vi "solar_app AppSetups (Dialog).vi"(11 "AppSetups":string[](array[string])) -> (3 "AppSetup":string)   [LabVIEW 2018]
doc: "This VI dialog selects the system setup to load for the application. Any setup other than \"Default\" adds a sub folder to the ..\\Configs folder. (i.e. \"Board\" Test Setup = ..\\Configs\\Board) All configuration files are kept in seperate folders for different system configurations."
panel:
  in  "Export":bool
  in  "OK":bool
  in  "Setup LB":i32(listbox)
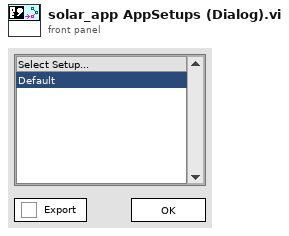
[diagram p1: front panel]
types:
  T1 = enum32{"invalid app kind", "Development System", "Run Time System", "Student Edition", "Embedded LabVIEW", "Evaluation", "Custom"}
  T2 = typedef "LVPoint32TypeDef.ctl" = cluster{"Horizontal":i32, "Vertical":i32}
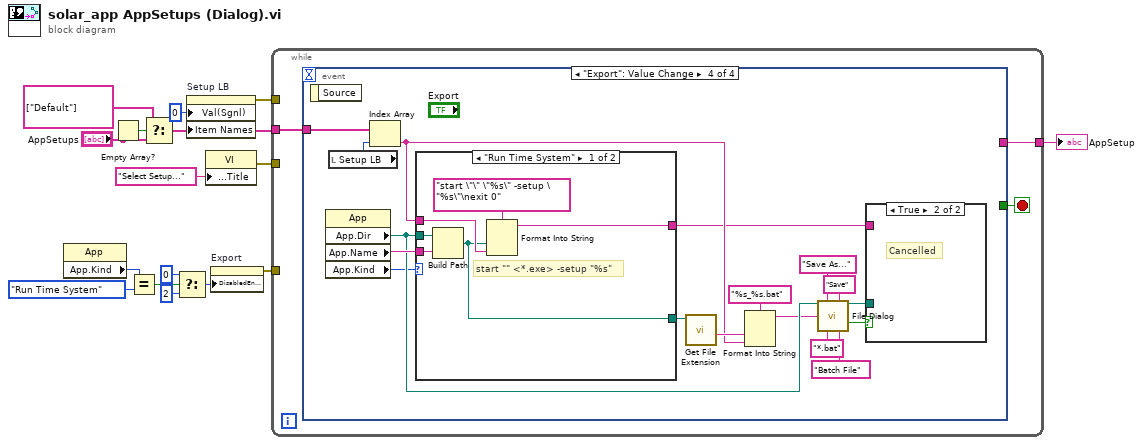
[diagram p0: block diagram]
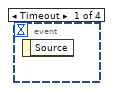
[diagram p2: hidden frame]
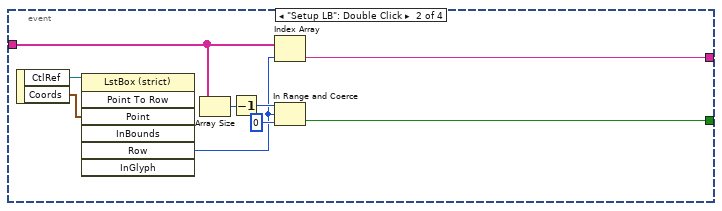
[diagram p3: hidden frame]
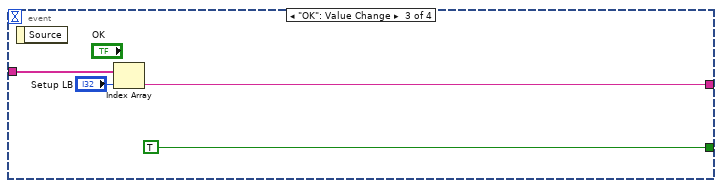
[diagram p4: hidden frame]
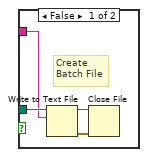
[diagram p5: hidden frame]
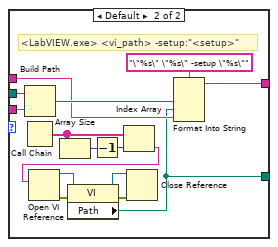
[diagram p6: hidden frame]
diagram:
  n1 = property class="App"() -> ("App.Kind"=w7:T1)  [unwired: 2 in, 2 out]
  n2 = Empty Array?(array="AppSetups") -> (empty?=w11:bool)
  n3 = Equal?(x=w7, y=T1."Run Time System") -> (x = y?=w5:bool)
  n4 = Select(t=string[] ["Default"], s=w11, f="AppSetups") -> (s? t:f=w8:string[])
  n5 = Select(t=u8 0, s=w5, f=u8 2) -> (s? t:f=w4:u8)
  n6 = property on="Setup LB" class="LstBox (strict)"("Val(Sgnl)"=0 ("Setup LB"), "Item Names"=w8) -> (error out=w16:errorcluster)  [unwired: 2 in, 1 out]
  n7 = property class="VI"("Front Panel.Title"="Select Setup..." ("Front Panel Window:Title")) -> (error out=w12:errorcluster)  [unwired: 2 in, 1 out]
  n8 = property on="Export" class="Bool"("DisabledEnum"=w4) -> (error out=w1:errorcluster)  [unwired: 2 in, 1 out]
  n9 = while {
    tunnel: w8 -> [w19]
    tunnel: w16 -> [_]
    tunnel: [w18] -> w15
    tunnel: w12 -> [_]
    tunnel: w1 -> [_]
    stop <- w17 stop-if-true
    n10 = event shown="[3] \"Export\": Value Change" {
      selector: _ -> [_ _ _ _]
      dyn-events: _ -> [_ _ _ _]
      timeout: _ -> [_ _ _ _]
      tunnel: w19 -> [_ w24 w31 w48]
      tunnel: [_ w28 w29 _] -> w18
      tunnel: [_ w25 TRUE _] -> w17
      event Timeout {
        n11 = event-data() -> ()  [unwired: 1 in, 1 out]
      }
      event "Setup LB": Double Click {
        n12 = event-data() -> ("CtlRef"=w27:refnum<vi>, "Coords"=w20:T2)  [unwired: 1 in]
        n13 = invoke class="LstBox (strict)" method="Point To Row"(reference=w27, "Point"=w20) -> ("Row"=w21:i32)  [unwired: 5 in, 6 out]
        n14 = Array Size(array=w24) -> (size(s)=w23:i32)
        n15 = Decrement(x=w23) -> (x-1=w22:i32)
        n16 = Index Array(array=w24, index=w21) -> (element=w28:string)
        n17 = In Range and Coerce(upper limit=w22, x=w21, lower limit=0) -> (In Range?=w25:bool)  [unwired: 1 out]
      }
      event "OK": Value Change {
        n18 = event-data() -> ()  [unwired: 1 in, 1 out]
        n19 = Index Array(array=w31, index="Setup LB") -> (element=w29:string)
      }
      event "Export": Value Change {
        n20 = event-data() -> ()  [unwired: 1 in, 1 out]
        n21 = property class="App"() -> ("App.Dir"=w46:path, "App.Name"=w49:string, "App.Kind"=w33:T1)  [unwired: 2 in, 2 out]
        n22 = local read "Setup LB"() -> (w47:i32)
        n23 = Index Array(array=w48, index=w47) -> (element=w39:string)
        n24 = case shown="\"Run Time System\"" w33 {
          tunnel: w46 -> [w59 w74]
          tunnel: w49 -> [w58 w73]
          tunnel: [w55 w62] -> w36
          tunnel: w39 -> [w56 w61]
          tunnel: [w54 w60] -> w41
          frame "Run Time System" {
            # "start \"\" <*.exe> -setup \"%s\""
            n25 = Build Path(base path=w59, name or relative path=w58) -> (appended path=w54:path)
            n26 = Format Into String(format string="start \"\" \"%s\" -setup \"%s\"\nexit 0", w54, w56) -> (resulting string=w55:string)  [unwired: 2 in, 1 out]
          }
          frame Default {
            # "<LabVIEW.exe> <vi_path> -setup:\"<setup>\""
            n27 = Build Path(base path=w74, name or relative path=w73) -> (appended path=w64:path)
            n28 = Call Chain() -> (call chain=w72:string[])
            n29 = Array Size(array=w72) -> (size(s)=w71:i32)
            n30 = Decrement(x=w71) -> (x-1=w70:i32)
            n31 = Index Array(array=w72, index=w70) -> (element=w69:string)
            n32 = Open VI Reference(vi path=w69) -> (vi reference=w67:refnum<vi>, error out=w68:errorcluster)  [unwired: 5 in]
            n33 = property class="VI"(reference=w67, error in=w68) -> (reference out=w65:refnum<vi>, error out=w66:errorcluster, "Path"=w60:path)
            n34 = Close Reference(reference=w65, error in (no error)=w66) -> ()  [unwired: 1 out]
            n35 = Format Into String(format string="\"%s\" \"%s\" -setup \"%s\"", w64, w60, w61) -> (resulting string=w62:string)  [unwired: 2 in, 1 out]
          }
        }
        n36 = call <vilib>:"Get File Extension.vi"("file"=w41) -> ("filename without extension"=w40:string)  [unwired: 6 in, 4 out]
        n37 = Format Into String(format string="%s_%s.bat", w40, w39) -> (resulting string=w37:string)  [unwired: 2 in, 1 out]
        n38 = call "File Dialog"("start path"=w46, "prompt"="Save As...", "button label"="Save", "default name"=w37, "pattern (all files)"="*.bat", "pattern label"="Batch File") -> ("selected path"=w34:path, "cancelled"=w35:bool)  [unwired: 6 in, 2 out]
        n39 = case shown="True" w35 {
          tunnel: w36 -> [w52 _]
          tunnel: w34 -> [w53 _]
          frame False {
            # "Create\nBatch File"
            n40 = Write to Text File(file (use dialog)=w53, text=w52) -> (refnum out=w51:refnum<file>, error out=w50:errorcluster)  [unwired: 2 in, 1 out]
            n41 = Close File(refnum=w51, error in=w50) -> ()  [unwired: 2 out]
          }
          frame True {
            # "Cancelled"
          }
        }
      }
    }
  }
  "AppSetup" <- w15
